vi "Read Result Queue.vi"(8 "error in (no error)":errorcluster, 11 "Test Executor in":refnum<class "Test Executor.lvclass">) -> (0 "error out":errorcluster, 2 "Result Queue":refnum<queue>, 3 "Test Executor out":refnum<class "Test Executor.lvclass">)   [LabVIEW 2017, in "Test Executor.lvclass"]
uses:
  Test Executor.lvclass
  Test Result/Test Result.lvclass
  Test Executor.lvclass/Test Executor.ctl
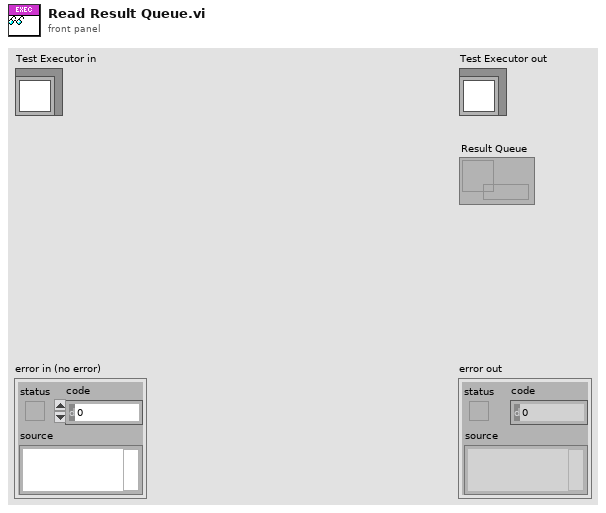
[diagram p1: front panel]
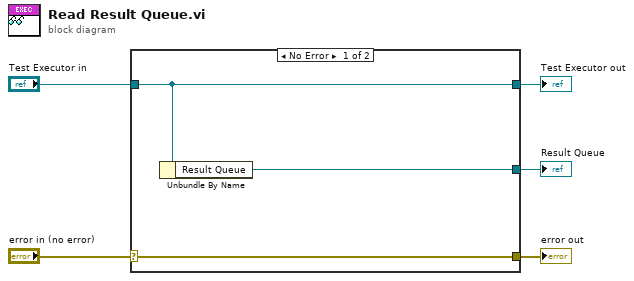
[diagram p0: block diagram]
diagram:
  n1 = case shown="No Error" "error in (no error)" {
    selector: "error in (no error)" -> [w8 w9]
    tunnel: [w8 w9] -> w4
    tunnel: [w7 w10] -> w2
    tunnel: "Test Executor in" -> [w7 w10]
    tunnel: [w6 _] -> w1
    frame No Error {
      n2 = Unbundle By Name(w7) -> ("Result Queue"=w6:refnum<queue>)
    }
    frame Error {
    }
  }
  "error out" <- w4
  "Test Executor out" <- w2
  "Result Queue" <- w1
